vi "configuration UI.vi"() -> ()   [LabVIEW 2013, in "fixed channel tag bus module editor node.lvclass"]
uses:
  fixed channel tag bus module editor node.lvclass
  <vilib>/CEF_TreeControl/Node/NodeRef.ctl
  <vilib>/CEF_TreeControl/Node/NISE_CEF_Node.lvclass
  <vilib>/NI/AMC/Message Queue.ctl
  <vilib>/NI/AMC/Message.ctl
  <vilib>/NI/Tools/Keyed Array/KeyedArray.ctl
  <vilib>/CEF_TreeControl/Node/UserEventRef.ctl
  <vilib>/CEF_TreeControl/Controls/EventCluster.ctl
  fixed channel tag bus module editor node.lvclass/fixed channel tag bus module editor node.ctl
  <vilib>/NI/Tag Bus Module Framework/root configuration/TBM configuration.lvclass/TBM configuration.ctl
  channel list helper functions.ctl
  <vilib>/NI/Tag Bus Module Framework/module configuration/TBM module configuration.lvclass
  <vilib>/NI/Tag Bus Module Framework/channel/TBM channel.lvclass
  <vilib>/NI/Tag Bus/tag/tag descriptor.lvclass/tag descriptor.ctl
  <vilib>/Utility/miscctls.llb/LVPoint32TypeDef.ctl
  <vilib>/NI/Tag Bus Module Framework/root configuration/Read instance name.vi
  <vilib>/NI/Tag Bus Module Framework/root configuration/create GUID.vi
  Configuration Editor/Classes/Module editor node/Read Module Configuration.vi
  <vilib>/NI/Module Execution Interface/Engine Configuration/engine configuration.lvclass
  <vilib>/NI/Tag Bus/tag/tag descriptor.lvclass
  <vilib>/CEF_TreeControl/NISE_CEF_TreeControl.lvlib
  Configuration Editor/Classes/Engine Parent/Engine Parent Editor Node.lvclass
  Configuration Editor/Classes/Module editor node/module editor node.lvclass
  module/configuration/fixed channel tag bus module configuration.lvclass
  <vilib>/NI/Tools/Keyed Array/Tools_KeyedArray.lvlib
  <vilib>/NI/AMC/AMC.lvlib
panel:
  out "Channel List":string[][](table)
  in  "user event":T1
  in  "main queue":T2
  in  "node ref":T3
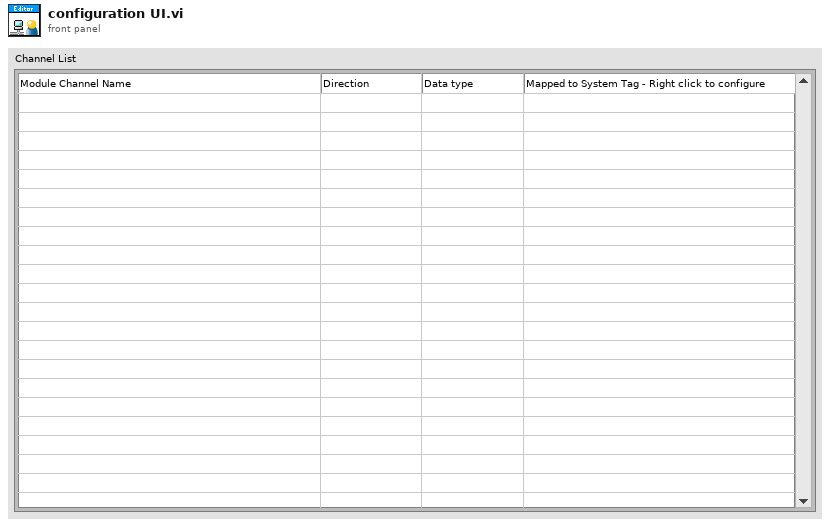
[diagram p1: front panel]
types:
  T1 = typedef "NISE_CEF_Node.lvclass/UserEventRef.ctl" = refnum<user-event>
  T2 = typedef "AMC.lvlib/Message Queue.ctl" = refnum<queue>
  T3 = typedef "NISE_CEF_Node.lvclass/NodeRef.ctl" = refnum<data-value>
  T4 = typedef "fixed channel tag bus module editor node.lvclass/channel list helper functions.ctl" = enum16{"Convert", "Get Value", "Update Value", "Analyze Table"}
  T5 = typedef "NISE_CEF_TreeControl.lvlib/EventCluster.ctl" = cluster{"command":string, "data":string}
  T6 = typedef "LVPoint32TypeDef.ctl" = cluster{"Horizontal":i32, "Vertical":i32}
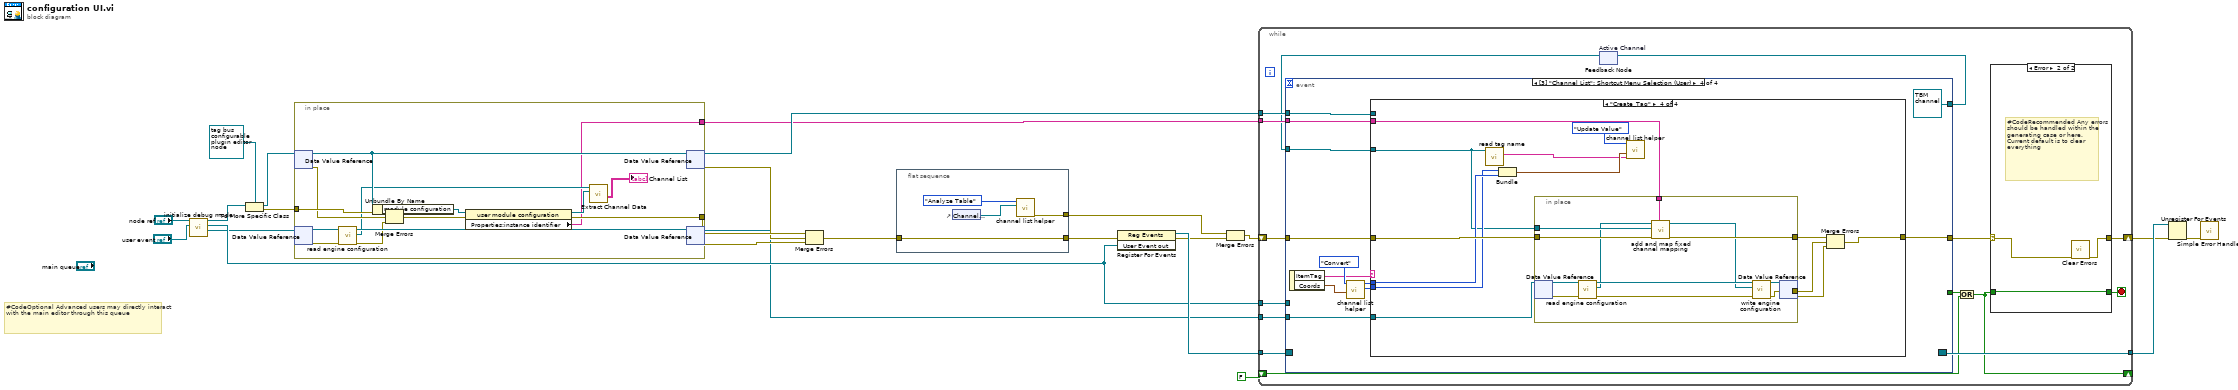
[diagram p0: block diagram]
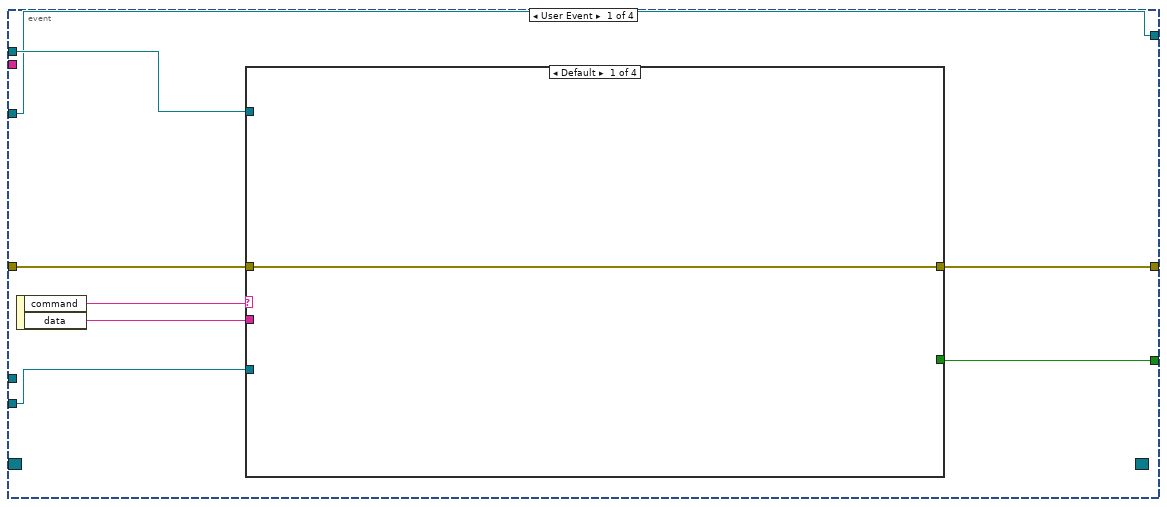
[diagram p3: hidden frame]
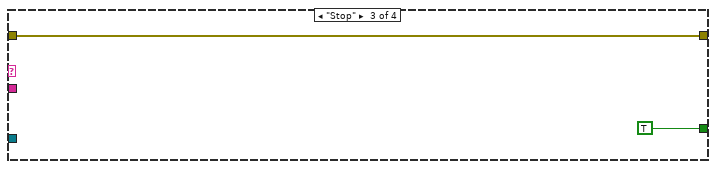
[diagram p5: hidden frame]
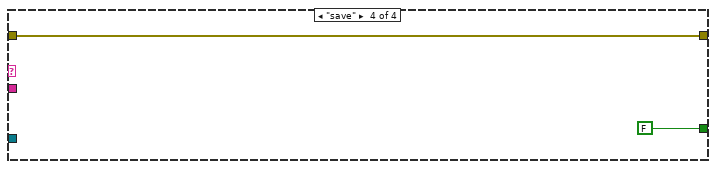
[diagram p6: hidden frame]
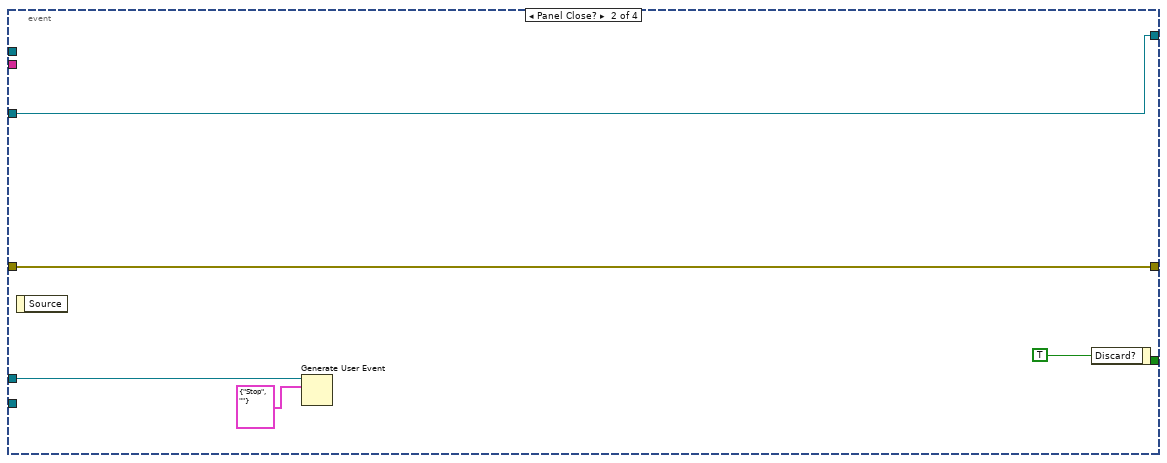
[diagram p7: hidden frame]
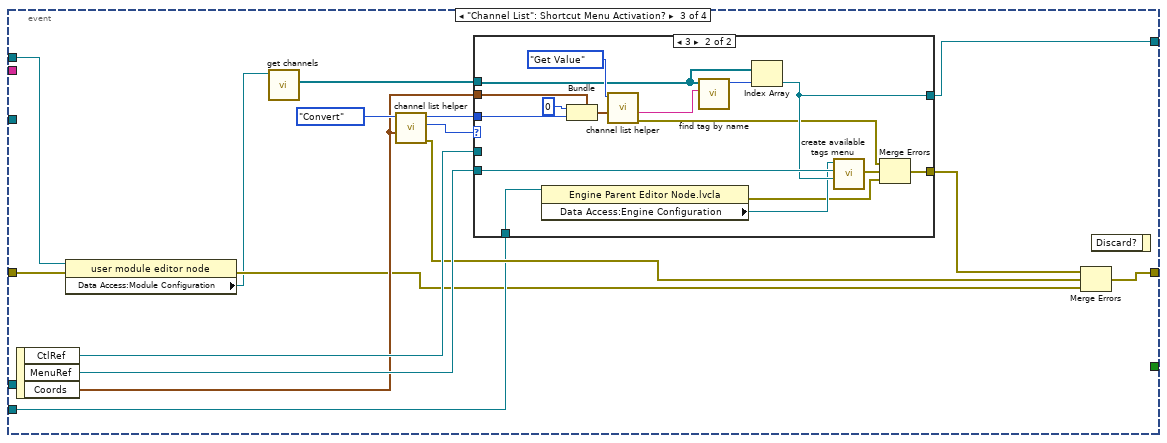
[diagram p8: hidden frame]
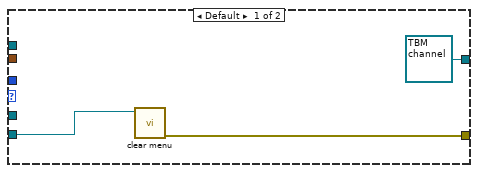
[diagram p9: hidden frame]
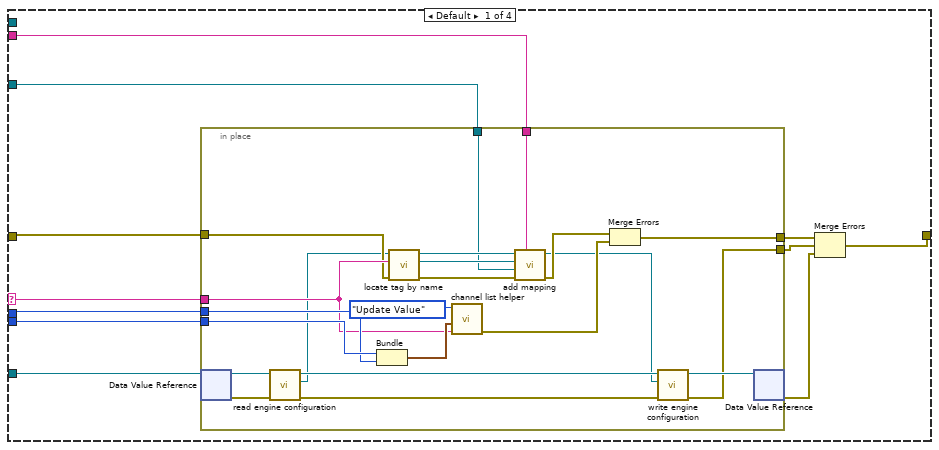
[diagram p10: hidden frame]
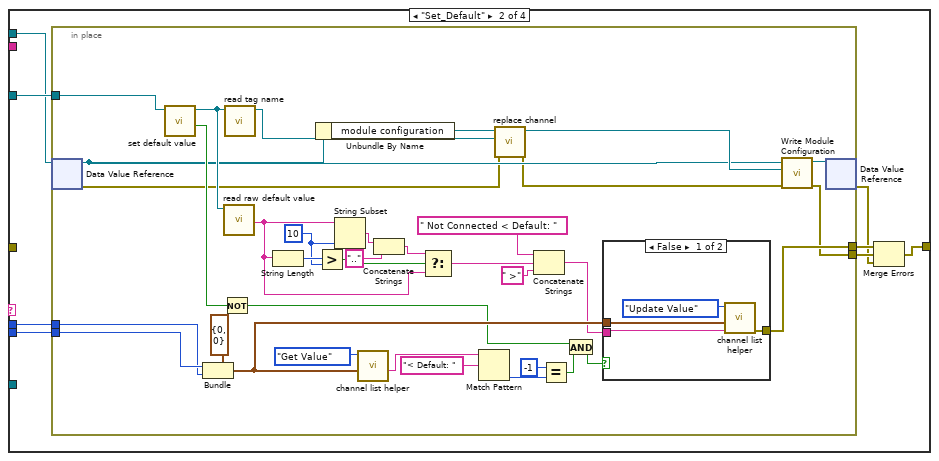
[diagram p11: hidden frame]
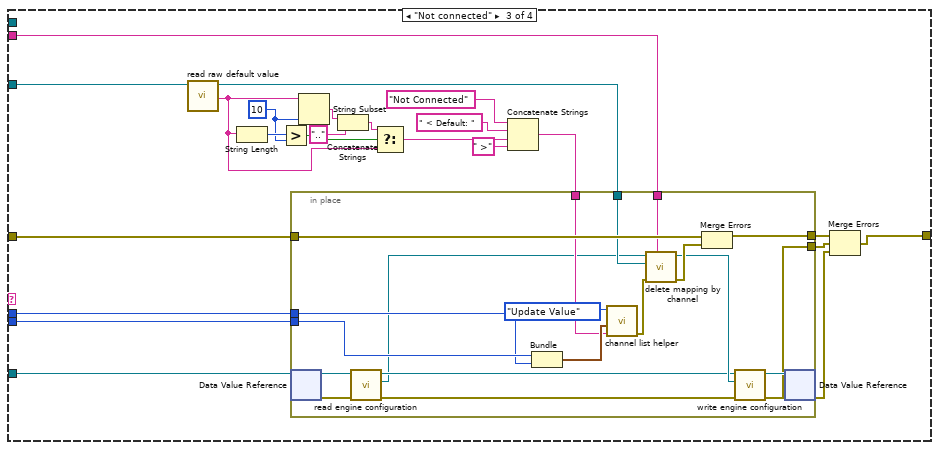
[diagram p13: hidden frame]
diagram:
  # "#CodeOptional Advanced users may directly interact with the main editor through this queue"
  n1 = call "initialize debug mode.vi"("User Event in"="user event", "editor node in"="node ref") -> ("engine"=w5:refnum<data-value>, "User Event out"=w12:T1, "editor node out"=w17:T3)  [unwired: 7 in]
  n2 = To More Specific Class(target class=refnum<data-value> refnum ("data value reference"), reference=w17) -> (specific class reference=w11:refnum<data-value>, error out=w9:errorcluster)  [unwired: 1 in]
  n3 = in-place {
    in-place-border: w9 -> [w38]
    in-place-border: [w30] -> w8
    in-place-border: [w27] -> w3
    n4 = in-place-dvr #1(w11) -> (w34:refnum<class "fixed channel tag bus module editor node.lvclass">, w37:errorcluster)
    n5 = in-place-dvr #2(w5) -> (w36:refnum<class "Engine Parent Editor Node.lvclass">, w25:errorcluster)
    n6 = call "read engine configuration.vi"("error in"=w25, "Engine Parent Editor Node in"=w36) -> ("error out"=w26:errorcluster, "engine configuration"=w32:refnum<class "engine configuration.lvclass">, "Engine Parent Editor Node out"=w35:refnum<class "Engine Parent Editor Node.lvclass">)  [unwired: 7 in]
    n7 = Unbundle By Name(w34) -> ("module configuration"=w29:refnum<class "fixed channel tag bus module configuration.lvclass">)
    n8 = Merge Errors(w38, w37, w26) -> (w33:errorcluster)
    n9 = property class="user module configuration"(reference=w29, error in=w33) -> (reference out=w28:refnum<class "fixed channel tag bus module configuration.lvclass">, error out=w30:errorcluster, "Properties:instance identifier"=w27:string)
    n10 = call "Extract Channel Data.vi"("module configuration"=w28, "Engine Configuration"=w32) -> ("Channel Data"=→"Channel List":string[][])  [unwired: 7 in, 2 out]
    n11 = in-place-dvr #1(w34) -> (w10:refnum<data-value>, w6:errorcluster)
    n12 = in-place-dvr #2(w35) -> (w4:refnum<data-value>, w7:errorcluster)
  }
  n13 = Merge Errors(w8, w6, w7) -> (w2:errorcluster)
  n14 = flat-sequence {
    tunnel: [w40] -> w13
    tunnel: w2 -> [w39]
    tunnel: [w39] -> w1
    frame #0 {
      n15 = control-ref of="Channel List"() -> (w42:refnum<vi>)
      n16 = call "channel list helper.vi"("Table In"=w42, "Function"=channel_list_helper_functions."Analyze Table") -> ("error out"=w40:errorcluster)  [unwired: 6 in, 3 out]
    }
  }
  n17 = register-events(error in=w1, w12) -> (reference out=w24:refnum<event-registration>, error out=w19:errorcluster)  [unwired: 1 in]
  n18 = Merge Errors(w13, w19) -> (w14:errorcluster)
  n19 = while {
    tunnel: w24 -> [w57]
    tunnel: [w56] -> w23
    shift-right: [w49] -> w22
    shift-left: w14 -> [w55]
    shift-right: [w51] -> _
    shift-left: FALSE -> [w50]
    tunnel: w3 -> [w48]
    tunnel: w10 -> [w47]
    tunnel: w4 -> [w46]
    tunnel: w12 -> [w43]
    stop <- w53 stop-if-true
    n20 = feedback #3 "Active Channel"() -> (w44:refnum<class "TBM channel.lvclass">)  [unwired: 1 in]
    n21 = event shown="[3] \"Channel List\": Shortcut Menu Selection (User)" {
      selector: w57 -> [_ _ _ _]
      dyn-events: [_ _ _ _] -> w56
      timeout: _ -> [_ _ _ _]
      tunnel: [w69 _ _ _] -> w52
      tunnel: [w70 w81 w92 w120] -> w54
      tunnel: w55 -> [w64 w81 w97 w121]
      tunnel: w48 -> [_ _ _ w119]
      tunnel: w47 -> [w67 _ w84 w117]
      tunnel: w46 -> [w66 _ w86 w118]
      tunnel: w44 -> [w63 w80 _ w122]
      tunnel: [w63 w80 w87 refnum<class "TBM channel.lvclass"> refnum ("channel")] -> w45
      tunnel: w43 -> [_ w78 _ _]
      event User Event {
        n22 = event-data() -> ("command"=w68:string, "data"=w65:string)  [unwired: 1 in]
        n23 = case shown="Default" w68 {
          tunnel: [_ _ TRUE FALSE] -> w69
          tunnel: w66 -> [_ _ _ _]
          tunnel: w64 -> [w71 w72 w73 w75]
          tunnel: [w71 w72 w73 w75] -> w70
          tunnel: w67 -> [_ _ _ _]
          tunnel: w65 -> [_ _ _ _]
          frame Default {
          }
          frame "Refresh" {
          }
          frame "Stop" {
          }
          frame "save" {
          }
        }
      }
      event Panel Close? {
        n24 = event-data() -> ()  [unwired: 1 in, 1 out]
        n25 = Generate User Event(user event=w78, event data cluster=T5 {"command"="Stop", "data"=""} ("event data")) -> ()  [unwired: 2 in, 2 out]
        n26 = event-data("Discard?"=TRUE) -> ()  [unwired: 1 in, 1 out]
      }
      event "Channel List": Shortcut Menu Activation? {
        n27 = event-data() -> ("CtlRef"=w90:refnum<vi>, "MenuRef"=w96:refnum<k9>, "Coords"=w89:T6)  [unwired: 1 in]
        n28 = property class="user module editor node"(reference=w84, error in=w97) -> (error out=w85:errorcluster, "Data Access:Module Configuration"=w83:refnum<class "TBM module configuration.lvclass">)  [unwired: 1 out]
        n29 = call-dynamic "get channels.vi"("module configuration in"=w83) -> ("channels"=w82:refnum<class "TBM channel.lvclass">[])  [unwired: 9 in, 1 out]
        n30 = call "channel list helper.vi"("Coords"=w89, "Function"=channel_list_helper_functions."Convert") -> ("error out"=w88:errorcluster, "Column"=w95:i32, "Row"=w94:i32)  [unwired: 6 in, 1 out]
        n31 = case shown="3" w95 {
          tunnel: w96 -> [w100 w116]
          tunnel: w94 -> [_ w111]
          tunnel: [w99 w105] -> w91
          tunnel: w90 -> [_ _]
          tunnel: w89 -> [_ w112]
          tunnel: w82 -> [_ w106]
          tunnel: [refnum<class "TBM channel.lvclass"> refnum ("channel") w110] -> w87
          tunnel: w86 -> [_ w103]
          frame Default {
            n32 = call "clear menu.vi"("Menu in"=w100) -> ("error out"=w99:errorcluster)  [unwired: 9 in, 1 out]
          }
          frame 3 {
            n33 = property class="Engine Parent Editor Node.lvcla"(reference=w103) -> (error out=w101:errorcluster, "Data Access:Engine Configuration"=w102:refnum<class "engine configuration.lvclass">)  [unwired: 1 in, 1 out]
            n34 = Bundle(cluster=w112, "Horizontal"=0, "Vertical"=w111) -> (w113:T6)
            n35 = call "channel list helper.vi"("Coords"=w113, "Function"=channel_list_helper_functions."Get Value") -> ("error out"=w104:errorcluster, "Value"=w108:string)  [unwired: 6 in, 2 out]
            n36 = call <vilib>:"find tag by name.vi"("name"=w108, "tags in"=w106) -> ("index"=w107:i32)  [unwired: 9 in]
            n37 = Index Array(array=w106, index=w107) -> (element=w110:refnum<class "TBM channel.lvclass">)
            n38 = call "create available tags menu.vi"("channel to map to"=w110, "MenuRef"=w116, "engine configuration in"=w102) -> ("error out"=w115:errorcluster)  [unwired: 7 in, 1 out]
            n39 = Merge Errors(w104, w115, w101) -> (w105:errorcluster)
          }
        }
        n40 = Merge Errors(w91, w88, w85) -> (w92:errorcluster)
        n41 = event-data() -> ()  [unwired: 2 in, 1 out]
      }
      event "Channel List": Shortcut Menu Selection (User) {
        n42 = event-data() -> ("ItemTag"=w124:string, "Coords"=w128:T6)  [unwired: 1 in]
        n43 = call "channel list helper.vi"("Coords"=w128, "Function"=channel_list_helper_functions."Convert") -> ("Column"=w127:i32, "Row"=w126:i32)  [unwired: 6 in, 2 out]
        n44 = case shown="\"Create_Tag\"" w124 {
          selector: w124 -> [w137 _ _ _]
          tunnel: w127 -> [w139 w168 w231 w257]
          tunnel: w126 -> [w138 w167 w230 w258]
          tunnel: w122 -> [w135 w169 w226 w252]
          tunnel: [w131 w164 w211 w255] -> w120
          tunnel: w121 -> [w136 _ w229 w263]
          tunnel: w119 -> [w133 _ w227 w261]
          tunnel: w118 -> [w132 _ w212 w256]
          tunnel: w117 -> [_ w165 _ _]
          frame Default {
            n45 = in-place {
              in-place-border: w139 -> [w160]
              in-place-border: w138 -> [w159]
              in-place-border: w137 -> [w157]
              in-place-border: w136 -> [w156]
              in-place-border: w135 -> [w153]
              in-place-border: [w150] -> w134
              in-place-border: w133 -> [w148]
              in-place-border: [w142] -> w129
              n46 = in-place-dvr #4(w132) -> (w145:refnum<class "Engine Parent Editor Node.lvclass">, w144:errorcluster)
              n47 = call "read engine configuration.vi"("error in"=w144, "Engine Parent Editor Node in"=w145) -> ("error out"=w146:errorcluster, "engine configuration"=w140:refnum<class "engine configuration.lvclass">, "Engine Parent Editor Node out"=w147:refnum<class "Engine Parent Editor Node.lvclass">)  [unwired: 7 in]
              n48 = Bundle("Column"=w160, "Row"=w159) -> (w158:cluster{"Column":i32, "Row":i32})  [unwired: 1 in]
              n49 = call <vilib>:"locate tag by name.vi"("error in"=w156, "tag name"=w157, "engine configuration in"=w140) -> ("error out"=w152:errorcluster, "tag descriptor"=w154:refnum<class "tag descriptor.lvclass">, "engine configuration out"=w155:refnum<class "engine configuration.lvclass">)  [unwired: 6 in]
              n50 = call "channel list helper.vi"("Value"=w157, "Coords"=w158, "Function"=channel_list_helper_functions."Update Value") -> ("error out"=w149:errorcluster)  [unwired: 5 in, 3 out]
              n51 = call <vilib>:"add mapping.vi"("owner ID"=w148, "error in"=w152, "channel"=w153, "tag descriptor"=w154, "engine configuration"=w155) -> ("error out"=w151:errorcluster, "engine configuration out"=w141:refnum<class "engine configuration.lvclass">)  [unwired: 5 in]
              n52 = Merge Errors(w151, w149) -> (w150:errorcluster)
              n53 = call "write engine configuration.vi"("error in"=w146, "engine configuration"=w141, "Engine Parent Editor Node in"=w147) -> ("error out"=w142:errorcluster, "Engine Parent Editor Node out"=w143:refnum<class "Engine Parent Editor Node.lvclass">)  [unwired: 7 in]
              n54 = in-place-dvr #4(w143) -> (w130:errorcluster)  [unwired: 1 out]
            }
            n55 = Merge Errors(w134, w129, w130) -> (w131:errorcluster)
          }
          frame "Set_Default" {
            n56 = in-place {
              in-place-border: w169 -> [w204]
              in-place-border: w168 -> [w203]
              in-place-border: w167 -> [w202]
              in-place-border: [w178] -> w166
              in-place-border: [w176] -> w163
              w187 = 10 ("y")
              n57 = in-place-dvr #5(w165) -> (w174:refnum<class "fixed channel tag bus module editor node.lvclass">, w172:errorcluster)
              n58 = call "set default value.vi"("tag"=w204) -> ("cancelled?"=w190:bool, "tag out"=w182:refnum<class "TBM channel.lvclass">)  [unwired: 9 in]
              n59 = Bundle(cluster=T6 {"Horizontal"=0, "Vertical"=0} ("Coords"), "Horizontal"=w203, "Vertical"=w202) -> (w194:T6)
              n60 = Not(x=w190) -> (.not. x?=w179:bool)
              n61 = call <vilib>:"read raw default value.vi"("system tag in"=w182) -> ("raw default"=w183:string)  [unwired: 8 in, 2 out]
              n62 = call <vilib>:"read tag name.vi"("system tag in"=w182) -> ("system tag out"=w170:refnum<class "TBM channel.lvclass">)  [unwired: 8 in, 2 out]
              n63 = String Length(string=w183) -> (length=w189:i32)
              n64 = Unbundle By Name(w174) -> ("module configuration"=w173:refnum<class "fixed channel tag bus module configuration.lvclass">)
              n65 = Greater?(x=w189, y=w187) -> (0:w188:bool)
              n66 = String Subset(string=w183, length (rest)=w187) -> (substring=w185:string)  [unwired: 1 in]
              n67 = call "channel list helper.vi"("Coords"=w194, "Function"=channel_list_helper_functions."Get Value") -> ("Value"=w199:string)  [unwired: 6 in, 3 out]
              n68 = Concatenate Strings(w185, ".." ("string")) -> (w186:string)
              n69 = Select(t=w186, s=w188, f=w183) -> (s? t:f=w181:string)
              n70 = Match Pattern(string=w199, regular expression="< Default: ") -> (offset past match=w197:i32)  [unwired: 1 in, 3 out]
              n71 = call "replace channel.vi"("error in"=w172, "channel"=w170, "user module configuration in"=w173) -> ("error out"=w171:errorcluster, "user module configuration out"=w175:refnum<class "fixed channel tag bus module configuration.lvclass">)  [unwired: 7 in]
              n72 = Concatenate Strings(" Not Connected < Default: " ("string"), w181, " >" ("string")) -> (w180:string)
              n73 = Equal?(x=-1, y=w197) -> (x = y?=w195:bool)
              n74 = And(x=w179, y=w195) -> (x .and. y?=w191:bool)
              n75 = case shown="False" w191 {
                tunnel: w194 -> [w207 _]
                tunnel: w180 -> [w206 _]
                tunnel: [w205 _] -> w178
                frame False {
                  n76 = call "channel list helper.vi"("Value"=w206, "Coords"=w207, "Function"=channel_list_helper_functions."Update Value") -> ("error out"=w205:errorcluster)  [unwired: 5 in, 3 out]
                }
                frame True {
                }
              }
              n77 = call "Write Module Configuration.vi"("error in"=w171, "module configuration"=w175, "Module Editor Node in"=w174) -> ("error out"=w176:errorcluster, "Module Editor Node out"=w177:refnum<class "fixed channel tag bus module editor node.lvclass">)  [unwired: 7 in]
              n78 = in-place-dvr #5(w177) -> (w162:errorcluster)  [unwired: 1 out]
            }
            n79 = Merge Errors(w166, w163, w162) -> (w164:errorcluster)
          }
          frame "Not connected" {
            w219 = 10 ("y")
            n80 = call <vilib>:"read raw default value.vi"("system tag in"=w226) -> ("raw default"=w215:string, "system tag out"=w225:refnum<class "TBM channel.lvclass">)  [unwired: 8 in, 1 out]
            n81 = String Length(string=w215) -> (length=w221:i32)
            n82 = Greater?(x=w221, y=w219) -> (0:w220:bool)
            n83 = String Subset(string=w215, length (rest)=w219) -> (substring=w217:string)  [unwired: 1 in]
            n84 = Concatenate Strings(w217, ".." ("string")) -> (w218:string)
            n85 = Select(t=w218, s=w220, f=w215) -> (s? t:f=w214:string)
            n86 = Concatenate Strings("Not Connected" ("string"), " < Default: " ("string"), w214, " >" ("string")) -> (w224:string)
            n87 = in-place {
              in-place-border: w231 -> [w249]
              in-place-border: w230 -> [w248]
              in-place-border: w229 -> [w245]
              in-place-border: [w244] -> w228
              in-place-border: w227 -> [w242]
              in-place-border: w225 -> [w241]
              in-place-border: w224 -> [w240]
              in-place-border: [w235] -> w209
              n88 = in-place-dvr #6(w212) -> (w239:refnum<class "Engine Parent Editor Node.lvclass">, w238:errorcluster)
              n89 = call "read engine configuration.vi"("error in"=w238, "Engine Parent Editor Node in"=w239) -> ("error out"=w236:errorcluster, "engine configuration"=w232:refnum<class "engine configuration.lvclass">, "Engine Parent Editor Node out"=w233:refnum<class "Engine Parent Editor Node.lvclass">)  [unwired: 7 in]
              n90 = Bundle("Column"=w249, "Row"=w248) -> (w247:cluster{"Column":i32, "Row":i32})  [unwired: 1 in]
              n91 = call "channel list helper.vi"("Value"=w240, "Coords"=w247, "Function"=channel_list_helper_functions."Update Value") -> ("error out"=w246:errorcluster)  [unwired: 5 in, 3 out]
              n92 = call <vilib>:"delete mapping by channel.vi"("owner ID"=w242, "error in"=w246, "channel"=w241, "engine configuration in"=w232) -> ("error out"=w243:errorcluster, "engine configuration out"=w234:refnum<class "engine configuration.lvclass">)  [unwired: 6 in]
              n93 = Merge Errors(w245, w243) -> (w244:errorcluster)
              n94 = call "write engine configuration.vi"("error in"=w236, "engine configuration"=w234, "Engine Parent Editor Node in"=w233) -> ("error out"=w235:errorcluster, "Engine Parent Editor Node out"=w237:refnum<class "Engine Parent Editor Node.lvclass">)  [unwired: 7 in]
              n95 = in-place-dvr #6(w237) -> (w210:errorcluster)  [unwired: 1 out]
            }
            n96 = Merge Errors(w228, w209, w210) -> (w211:errorcluster)
          }
          frame "Create_Tag" {
            n97 = call <vilib>:"read tag name.vi"("system tag in"=w252) -> ("name"=w251:string)  [unwired: 8 in, 2 out]
            n98 = Bundle("Column"=w257, "Row"=w258) -> (w259:cluster{"Column":i32, "Row":i32})  [unwired: 1 in]
            n99 = in-place {
              in-place-border: w263 -> [w275]
              in-place-border: [w274] -> w262
              in-place-border: w261 -> [w273]
              in-place-border: w252 -> [w272]
              in-place-border: [w268] -> w253
              n100 = in-place-dvr #7(w256) -> (w270:refnum<class "Engine Parent Editor Node.lvclass">, w271:errorcluster)
              n101 = call "read engine configuration.vi"("error in"=w271, "Engine Parent Editor Node in"=w270) -> ("error out"=w267:errorcluster, "engine configuration"=w265:refnum<class "engine configuration.lvclass">, "Engine Parent Editor Node out"=w266:refnum<class "Engine Parent Editor Node.lvclass">)  [unwired: 7 in]
              n102 = call <vilib>:"add and map fixed channel mapping.vi"("module instance"=w273, "error in"=w275, "fixed channel"=w272, "engine configuration in"=w265) -> ("error out"=w274:errorcluster, "engine configuration out"=w264:refnum<class "engine configuration.lvclass">)  [unwired: 6 in]
              n103 = call "write engine configuration.vi"("error in"=w267, "engine configuration"=w264, "Engine Parent Editor Node in"=w266) -> ("error out"=w268:errorcluster, "Engine Parent Editor Node out"=w269:refnum<class "Engine Parent Editor Node.lvclass">)  [unwired: 7 in]
              n104 = in-place-dvr #7(w269) -> (w254:errorcluster)  [unwired: 1 out]
            }
            n105 = call "channel list helper.vi"("Value"=w251, "Coords"=w259, "Function"=channel_list_helper_functions."Update Value") -> ()  [unwired: 5 in, 4 out]
            n106 = Merge Errors(w262, w253, w254) -> (w255:errorcluster)
          }
        }
      }
    }
    n107 = feedback-in #3(w45) -> ()
    n108 = Or(x=w52, y=w50) -> (x .or. y?=w51:bool)
    n109 = case shown="Error" w54 {
      selector: w54 -> [w58 w60]
      tunnel: [w59 w62] -> w53
      tunnel: w51 -> [w59 w62]
      tunnel: [w58 w61] -> w49
      frame No Error {
      }
      frame Error {
        # "#CodeRecommended Any errors should be handled within the generating case or here. Current default is to clear everything"
        n110 = call <vilib>:"Clear Errors.vi"("error in (no error)"=w60) -> ("error out"=w61:errorcluster)  [unwired: 6 in]
      }
    }
  }
  n111 = Unregister For Events(event registration refnum=w23, error in=w22) -> (error out=w18:errorcluster)
  n112 = call <vilib>:"Simple Error Handler.vi"("error in (no error)"=w18) -> ()  [unwired: 4 in, 5 out]
